vi "svx_SC Line Event Consumer.vi"(7 "shaft centerline":T2, 8 "State in":T3={"X Scale"={"Name"="Horizontal", "format string"="%#.2g", "Major Color"=16777238, "Minor Color"=16777216, "Scale Visible"=TRUE, " Label Visible"=TRUE, "Grid Style"=1, "Maximum"=1.0, "Minimum"=-1.0}, "Y Scale"={"Name"="Vertical", "format string"="%#.2g", "Major Color"=16777238, "Minor Color"=16777216, "Scale Visible"=TRUE, " Label Visible"=TRUE, "Grid Style"=1, "Maximum"=1.0, "Minimum"=-1.0}, "Plot"={"Point Style"=0, "Line Width"=0, "Line Style"=0, "Plot Color"=16860, "Point/fill"=16860}, "Arrow Color"=16860, "Autoscale"=TRUE, "Property Name"=[], "Container Bounds"={"Width"=550, "Height"=313}, "Background color"=16777226, "Annotation List"=[], "Cursor"={"Cursor Point Style"=13, "Cursor Style"=4, "Cursor Line Width"=1, "Cursor Line Style"=0, "Cursor Color"=16711680, "Cursor Name Visible"=TRUE, "Cursor Visible"=TRUE, "Cursor Position"={"X"=0.0, "Y"=0.0}, "Cursor Index"=0, "Lock Cursor Name"=FALSE, "Cursor reference"=0.0}, "size"=0, "Boundary Color"=9868950, "Maximum"=1.0, "Marker Point Style"=2, "Maker Visible"=TRUE, "Marker Color"=16860, "pair strings []"=[], "clearance boundary"=[{"boundary"={"x axis"=0.0, "y axis"=0.0}, "start point"=enum."center"}], "Custom pair name"=FALSE, "selector.visible"=TRUE, "Cursor Release"=refnum, "Children Tags"=[], "open?"=TRUE, "pair index"=[], "Legend Width"=200, " Parents Tags"="", "Label"="", "Legend Background"=16777226, "Legend Font"=16777222, "scale fit"=2, "user strings []"=[], "Item Width"=0, "out of state queue"=refnum, "property nodes"=refnum, "Kind"=enum."X-Scale", "Scale Range Change"=refnum} caption="State" {"pair index" min=0}, 10 "events":T7[](array[typedef]), 11 "references":T1) -> (0 "State out":T3={"X Scale"={"Name"="Horizontal", "format string"="%#.2g", "Major Color"=16777238, "Minor Color"=16777216, "Scale Visible"=TRUE, " Label Visible"=TRUE, "Grid Style"=1, "Maximum"=1.0, "Minimum"=-1.0}, "Y Scale"={"Name"="Vertical", "format string"="%#.2g", "Major Color"=16777238, "Minor Color"=16777216, "Scale Visible"=TRUE, " Label Visible"=TRUE, "Grid Style"=1, "Maximum"=1.0, "Minimum"=-1.0}, "Plot"={"Point Style"=0, "Line Width"=0, "Line Style"=0, "Plot Color"=16860, "Point/fill"=16860}, "Arrow Color"=16860, "Autoscale"=TRUE, "Property Name"=[], "Container Bounds"={"Width"=550, "Height"=313}, "Background color"=16777226, "Annotation List"=[], "Cursor"={"Cursor Point Style"=13, "Cursor Style"=4, "Cursor Line Width"=1, "Cursor Line Style"=0, "Cursor Color"=16711680, "Cursor Name Visible"=TRUE, "Cursor Visible"=TRUE, "Cursor Position"={"X"=0.0, "Y"=0.0}, "Cursor Index"=0, "Lock Cursor Name"=FALSE, "Cursor reference"=0.0}, "size"=0, "Boundary Color"=9868950, "Maximum"=1.0, "Marker Point Style"=2, "Maker Visible"=TRUE, "Marker Color"=16860, "pair strings []"=[], "clearance boundary"=[{"boundary"={"x axis"=0.0, "y axis"=0.0}, "start point"=enum."center"}], "Custom pair name"=FALSE, "selector.visible"=TRUE, "Cursor Release"=refnum, "Children Tags"=[], "open?"=TRUE, "pair index"=[], "Legend Width"=200, " Parents Tags"="", "Label"="", "Legend Background"=16777226, "Legend Font"=16777222, "scale fit"=2, "user strings []"=[], "Item Width"=0, "out of state queue"=refnum, "property nodes"=refnum, "Kind"=enum."X-Scale", "Scale Range Change"=refnum} caption="State" {"pair index" min=0})   [LabVIEW 2017, in "SVX SC Line.xctl"]
uses:
  <vilib>/addons/_XControls/Shaft Centerline/SVX SC Line.xctl
  <vilib>/addons/_XControls/Shaft Centerline/subVIs/svx_SC Line Core States.ctl
  <vilib>/addons/_XControls/Shaft Centerline/subVIs/svx_SC Line State.ctl
  <vilib>/addons/_XControls/Shaft Centerline/subVIs/svx_SC Line Bounds.ctl
  <vilib>/addons/_XControls/Shaft Centerline/subVIs/svx_SC Line Annotation List.ctl
  <vilib>/addons/_XControls/Shaft Centerline/subVIs/svx_SC Line OutState Queue.ctl
  <vilib>/addons/_XControls/Shaft Centerline/subVIs/svx_SC Line Data.ctl
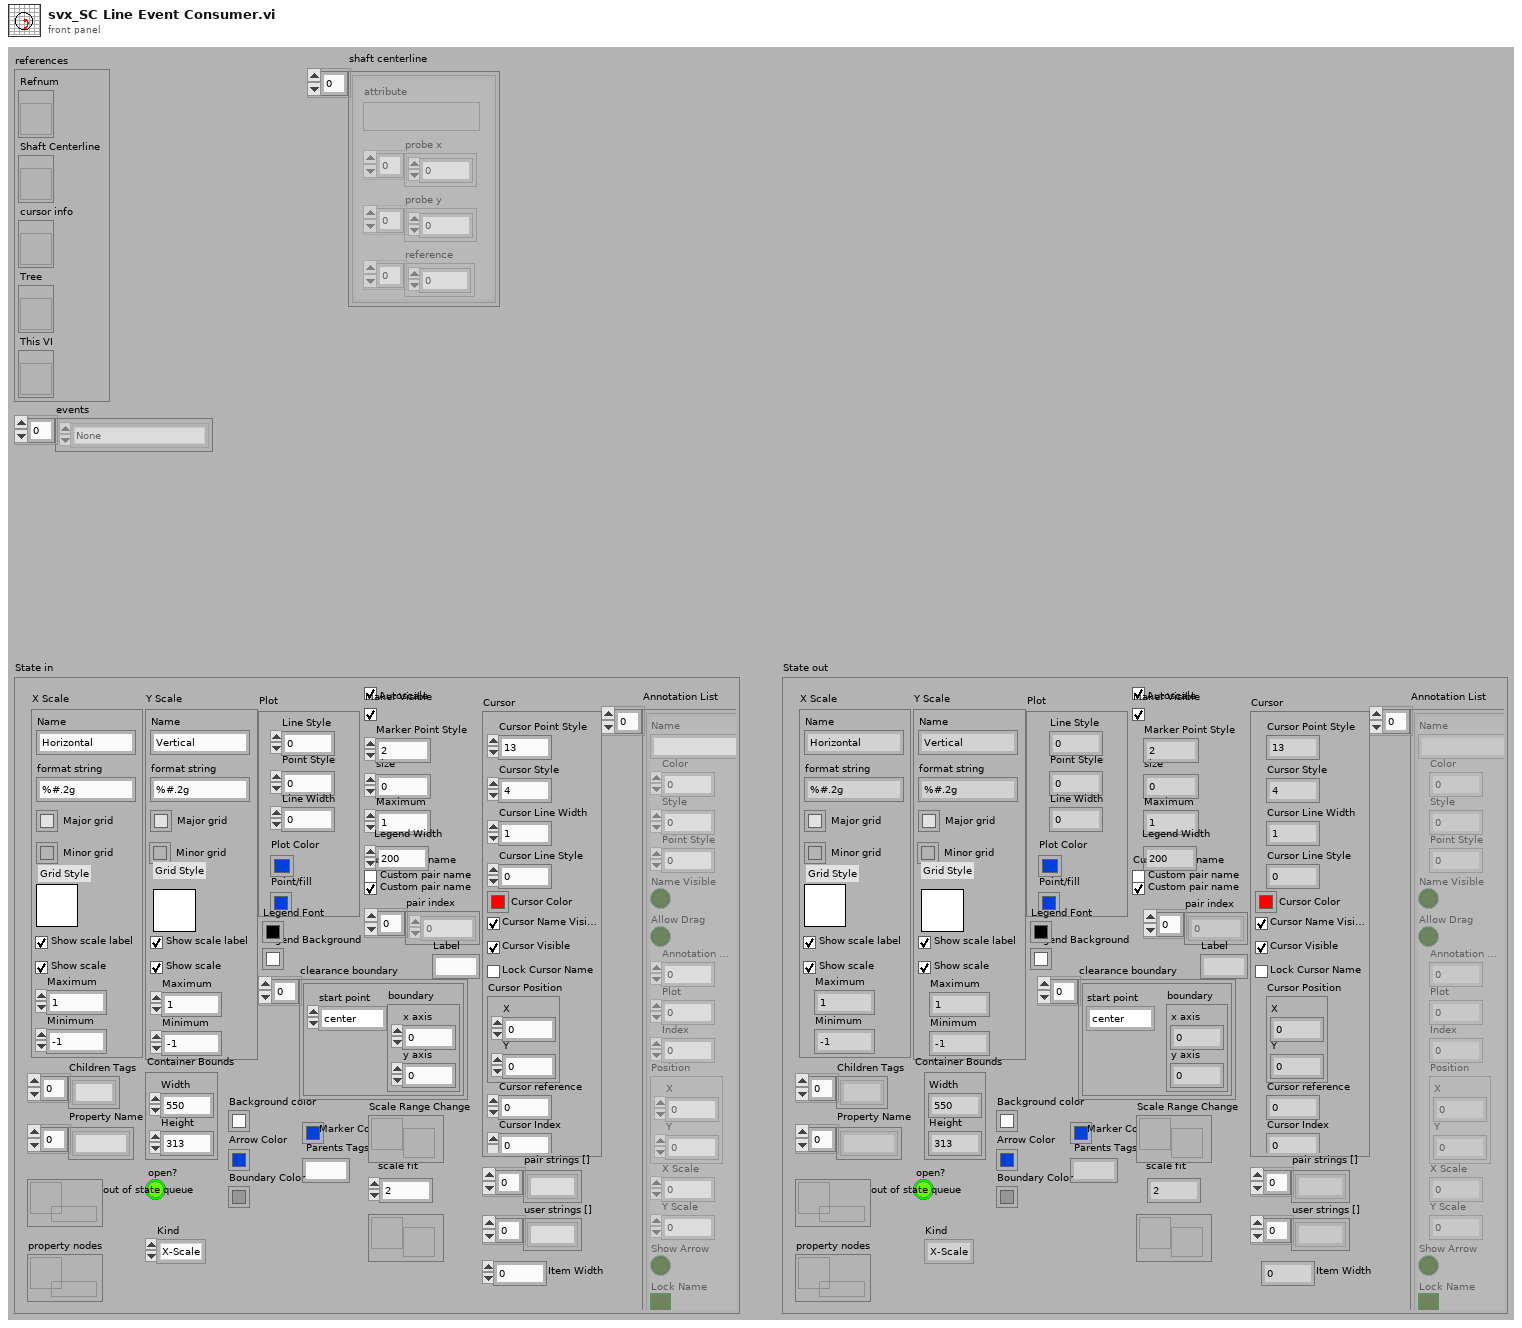
[diagram p1: front panel]
types:
  T1 = cluster{"Refnum":refnum<vi>, "Shaft Centerline":refnum<vi>, "cursor info":refnum<vi>, "Tree":refnum<vi>, "This VI":refnum<vi>}
  T2 = typedef "SVX SC Line.xctl/svx_SC Line Data.ctl" = cluster{"probe x":dbl[], "probe y":dbl[], "reference":dbl[], "attribute":variant}[]
  T3 = typedef "SVX SC Line.xctl/svx_SC Line State.ctl" = cluster{"X Scale":cluster{"Name":string, "format string":string, "Major Color":u32, "Minor Color":u32, "Scale Visible":bool, " Label Visible":bool, "Grid Style":u16, "Maximum":dbl, "Minimum":dbl}, "Y Scale":cluster{"Name":string, "format string":string, "Major Color":u32, "Minor Color":u32, "Scale Visible":bool, " Label Visible":bool, "Grid Style":u16, "Maximum":dbl, "Minimum":dbl}, "Plot":cluster{"Point Style":u8, "Line Width":u8, "Line Style":u8, "Plot Color":u32, "Point/fill":u32}, "Arrow Color":u32, "Autoscale":bool, "Property Name":string[], "Container Bounds":T4, "Background color":u32, "Annotation List":T5, "Cursor":cluster{"Cursor Point Style":u8, "Cursor Style":u8, "Cursor Line Width":u8, "Cursor Line Style":u8, "Cursor Color":u32, "Cursor Name Visible":bool, "Cursor Visible":bool, "Cursor Position":cluster{"X":dbl, "Y":dbl}, "Cursor Index":i32, "Lock Cursor Name":bool, "Cursor reference":dbl}, "size":i32, "Boundary Color":u32, "Maximum":dbl, "Marker Point Style":u8, "Maker Visible":bool, "Marker Color":u32, "pair strings []":string[], "clearance boundary":cluster{"boundary":cluster{"x axis":dbl, "y axis":dbl}, "start point":enum16{"center", "top", "bottom"}}[], "Custom pair name":bool, "selector.visible":bool, "Cursor Release":refnum<user-event>, "Children Tags":string[], "open?":bool, "pair index":i32[], "Legend Width":u32, " Parents Tags":string, "Label":string, "Legend Background":u32, "Legend Font":u32, "scale fit":u8, "user strings []":string[], "Item Width":u32, "out of state queue":T6, "property nodes":refnum<queue>, "Kind":enum16{"X-Scale", "Y-Scale", "Z-Scale"}, "Scale Range Change":refnum<user-event>}
  T4 = typedef "SVX SC Line.xctl/svx_SC Line Bounds.ctl" = cluster{"Width":u32, "Height":u32}
  T5 = typedef "SVX SC Line.xctl/svx_SC Line Annotation List.ctl" = cluster{"Name":string, "Color":u32, "Style":u8, "Point Style":u8, "Name Visible":bool, "Allow Drag":bool, "Annotation Mode":u32, "Plot":i32, "Index":i32, "Position":cluster{"X":dbl, "Y":dbl}, "X Scale":u32, "Y Scale":u32, "Show Arrow":bool, "Lock Name":bool, "Plot Area":i32, "Label Offset":cluster{"X":dbl, "Y":dbl}}[]
  T6 = typedef "SVX SC Line.xctl/svx_SC Line OutState Queue.ctl" = refnum<queue>
  T7 = typedef "SVX SC Line.xctl/svx_SC Line Core States.ctl" = enum16{"None", "[Axis] Autoscale", "[Image] Update", "[Cursor] Name", "[Plot] Grid&BG", "[Marker] Update", "[Tree] Tags", "[Data] Update", "[Layout] Size", "[Tree] Checkbox", "[Tree] Visible", "[Tree] Open", "[Axis] X", "[Axis] Y", "[Plot] Color", "[Axis] Format String", "[Data] Compare Strings", "[Cursor] Apearance", "[Axis] Name&Visible", "[Tree] Color", "[Data] Index", "[Cursor] Index", "[Axis] Event"}
  T8 = cluster{"X.Minimum":dbl, "X.Maximum":dbl, "Y.Minimum":dbl, "Y.Maximum":dbl, "Kind":enum16{"X-Scale", "Y-Scale", "Z-Scale"}}
  T9 = cluster{"boundary":cluster{"x axis":dbl, "y axis":dbl}, "start point":enum16{"center", "top", "bottom"}}[]
  T10 = cluster{"probe x":dbl[], "probe y":dbl[], "reference":dbl[], "attribute":variant}
  T11 = cluster{"boundary":cluster{"x axis":dbl, "y axis":dbl}, "start point":enum16{"center", "top", "bottom"}}
  T12 = cluster{"Cursor Point Style":u8, "Cursor Style":u8, "Cursor Line Width":u8, "Cursor Line Style":u8, "Cursor Color":u32, "Cursor Name Visible":bool, "Cursor Visible":bool, "Cursor Position":cluster{"X":dbl, "Y":dbl}, "Cursor Index":i32, "Lock Cursor Name":bool, "Cursor reference":dbl}
  T13 = typedef "LVPointDoubleTypeDef.ctl" = cluster{"Cursor X":dbl, "Cursor Y":dbl}
  T14 = cluster{"use queue?":bool, "Legend Width":u32, "Cursor reference":dbl, "Cursor Position":cluster{"X":dbl, "Y":dbl}, "pair strings []":string[], "Label":string, "Parents Tags":string, "Children Tags":string[], "Item Width":u32, "Maximum":dbl, "Minimum":dbl, "Maximum":dbl, "Minimum":dbl, "selector.visible":bool, "clearance boundary":cluster{"boundary":cluster{"x axis":dbl, "y axis":dbl}, "start point":enum16{"center", "top", "bottom"}}[], "size":i32}
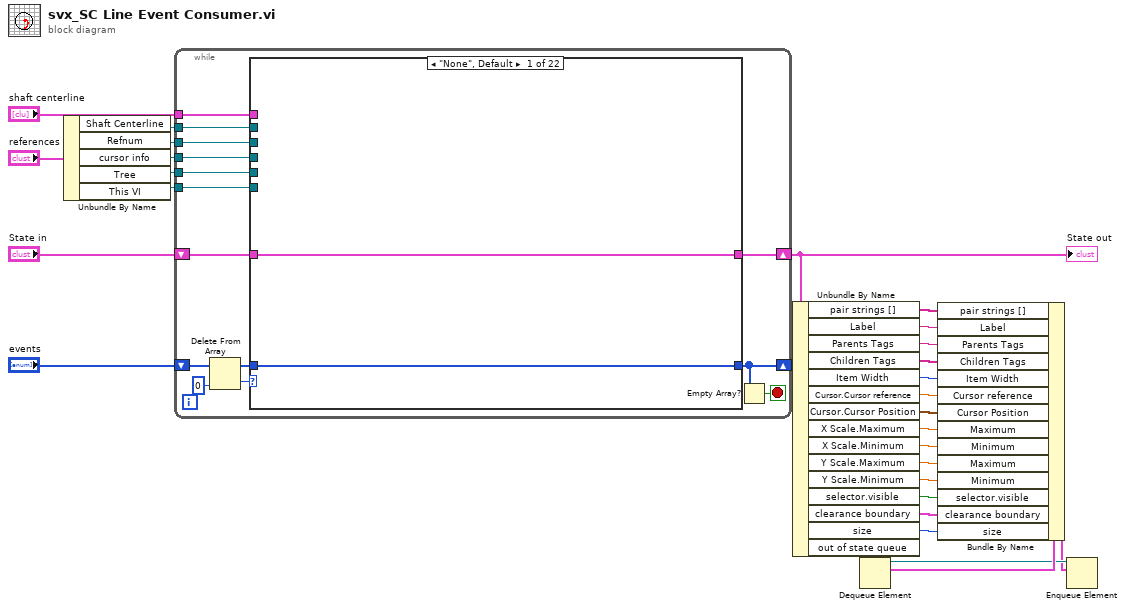
[diagram p0: block diagram]
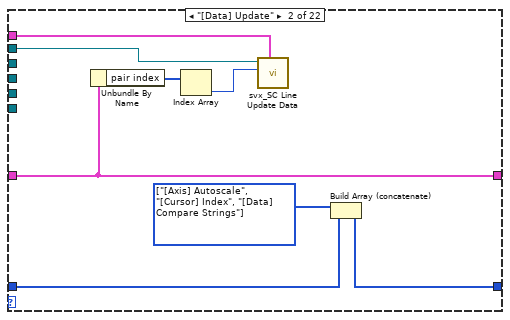
[diagram p2: hidden frame]
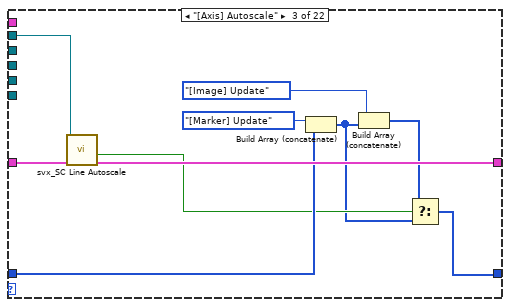
[diagram p3: hidden frame]
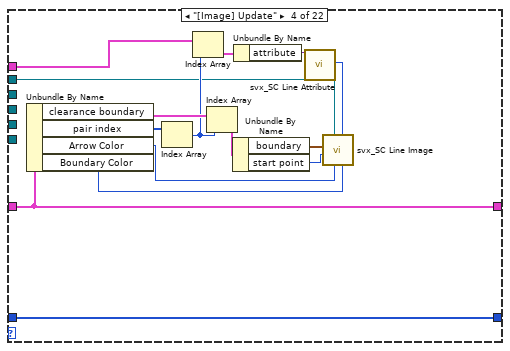
[diagram p4: hidden frame]
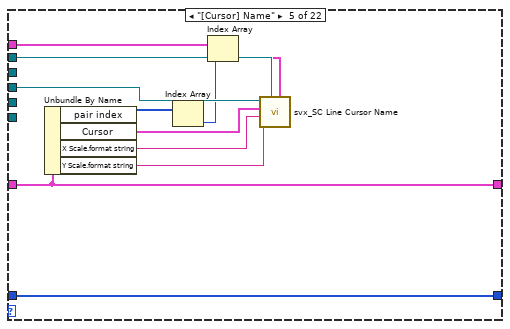
[diagram p5: hidden frame]
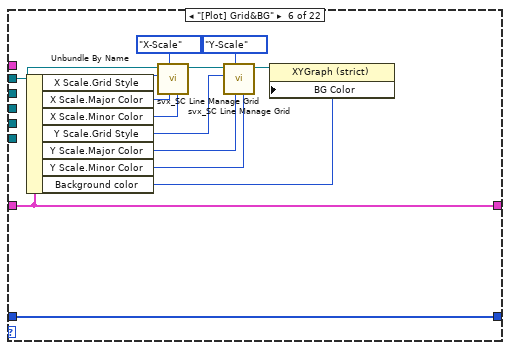
[diagram p6: hidden frame]
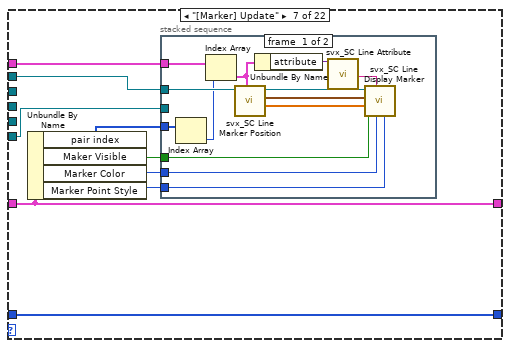
[diagram p7: hidden frame]
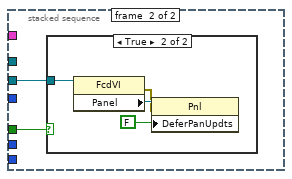
[diagram p8: hidden frame]
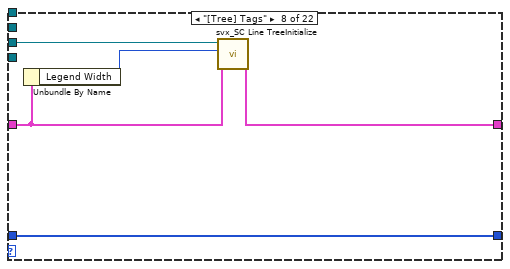
[diagram p10: hidden frame]
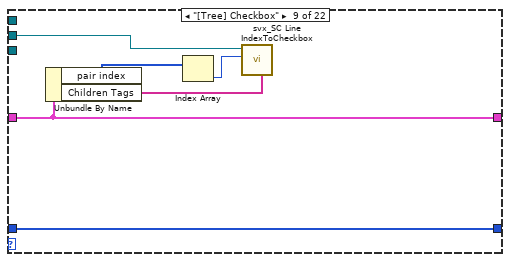
[diagram p11: hidden frame]
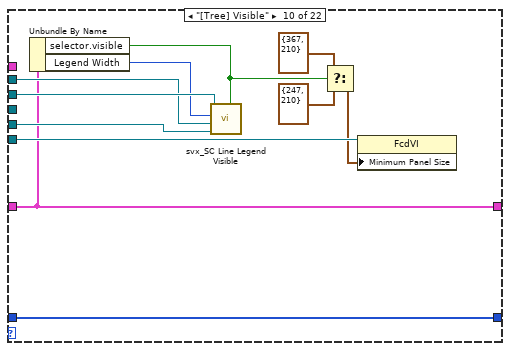
[diagram p12: hidden frame]
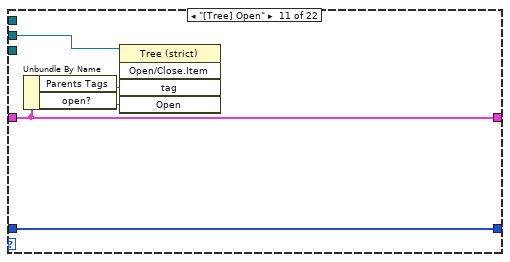
[diagram p13: hidden frame]
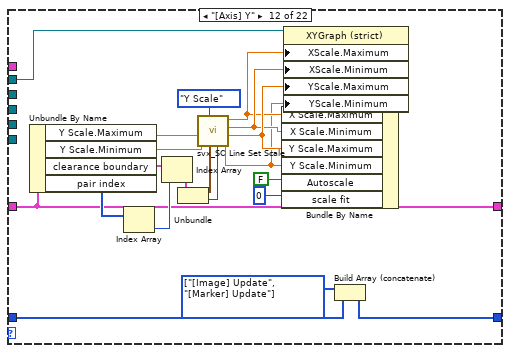
[diagram p14: hidden frame]
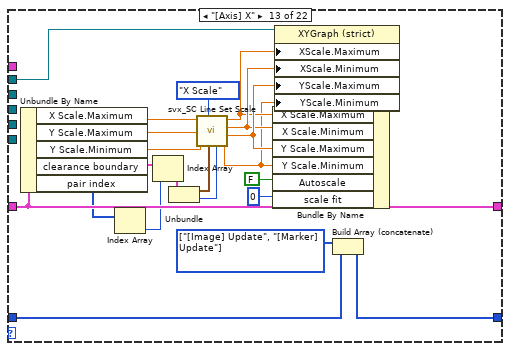
[diagram p15: hidden frame]
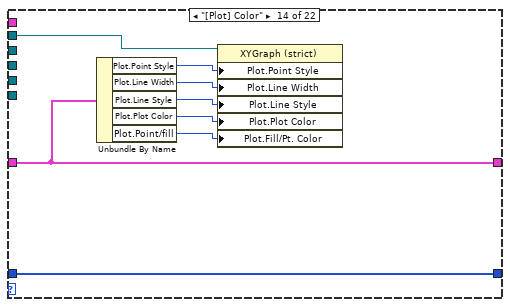
[diagram p16: hidden frame]
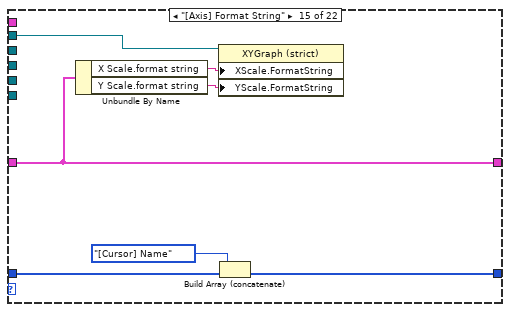
[diagram p17: hidden frame]
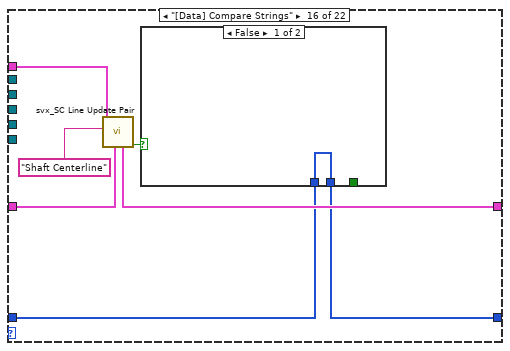
[diagram p18: hidden frame]
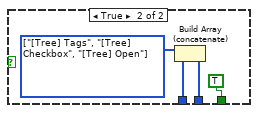
[diagram p19: hidden frame]
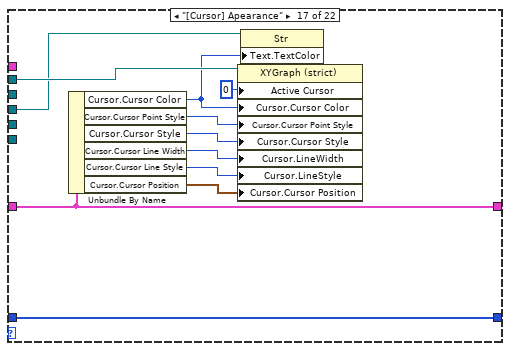
[diagram p20: hidden frame]
diagram:
  n1 = Unbundle By Name("references") -> ("Shaft Centerline"=w26:refnum<vi>, "Refnum"=w23:refnum<vi>, "cursor info"=w25:refnum<vi>, "Tree"=w24:refnum<vi>, "This VI"=w21:refnum<vi>)
  n2 = while {
    shift-right: [w42] -> w8
    shift-left: "State in" -> [w30]
    shift-right: [w36] -> _
    shift-left: "events" -> [w41]
    tunnel: "shaft centerline" -> [w35]
    tunnel: w26 -> [w34]
    tunnel: w25 -> [w33]
    tunnel: w24 -> [w32]
    tunnel: w23 -> [w31]
    tunnel: w21 -> [w29]
    stop <- w37 stop-if-true
    n3 = Delete From Array(array=w41, index=0) -> (deleted portion=w39:T7, array with subset deleted=w38:T7[])  [unwired: 1 in]
    n4 = case shown="\"None\", Default" w39 {
      tunnel: [w44 w50 w61 w77 w88 w93 w110 w135 w140 w142 w153 w166 w194 w202 w212 w221 w231 w247 w249 w264 w284 w292] -> w42
      tunnel: w38 -> [w43 w46 w58 w64 w78 w91 w104 w133 w136 w149 w154 w160 w181 w201 w210 w219 w230 w239 w248 w256 w286 w291]
      tunnel: [w43 w45 w59 w64 w78 w91 w104 w133 w136 w149 w154 w159 w180 w201 w209 w218 w230 w239 w248 w255 w285 w291] -> w36
      tunnel: w35 -> [_ w52 _ w67 w80 _ w105 _ _ _ _ _ _ _ _ w220 _ _ _ w274 _ _]
      tunnel: w34 -> [_ w51 w60 w63 w84 w92 w107 _ _ w151 _ w163 w192 w208 w215 _ w237 w246 _ w269 _ _]
      tunnel: w33 -> [_ _ _ _ w83 _ _ _ _ _ _ _ _ _ _ _ w229 _ _ _ _ _]
      tunnel: w32 -> [_ _ _ _ _ _ _ w134 w137 w150 w157 _ _ _ _ _ _ _ w252 _ _ _]
      tunnel: w31 -> [_ _ _ _ _ _ _ _ _ w152 _ _ _ _ _ _ _ _ _ _ _ _]
      tunnel: w30 -> [w44 w50 w62 w77 w88 w93 w110 w132 w140 w142 w153 w165 w193 w202 w212 w222 w231 w247 w249 w265 w284 w292]
      tunnel: w29 -> [_ _ _ _ _ _ w103 _ _ w146 _ _ _ _ _ _ _ _ _ _ _ _]
      frame "None", Default {
      }
      frame "[Data] Update" {
        w47 = T7[] [enum."[Axis] Autoscale", enum."[Cursor] Index", enum."[Data] Compare Strings"] items=["None", "[Axis] Autoscale", "[Image] Update", "[Cursor] Name", "[Plot] Grid&BG", "[Marker] Update", "[Tree] Tags", "[Data] Update", "[Layout] Size", "[Tree] Checkbox", "[Tree] Visible", "[Tree] Open", "[Axis] X", "[Axis] Y", "[Plot] Color", "[Axis] Format String", "[Data] Compare Strings", "[Cursor] Apearance", "[Axis] Name&Visible", "[Tree] Color", "[Data] Index", "[Cursor] Index", "[Axis] Event"] ("array")
        n5 = Unbundle By Name(w50) -> ("pair index"=w49:i32[])
        n6 = Index Array(array=w49) -> (element=w48:i32)  [unwired: 1 in]
        n7 = call <vilib>:"svx_SC Line Update Data.vi"("shaft centerline"=w52, "index"=w48, "reference"=w51) -> ()  [unwired: 9 in]
        n8 = Build Array (concatenate)(w47, w46) -> (w45:T7[])
      }
      frame "[Axis] Autoscale" {
        n9 = call <vilib>:"svx_SC Line Autoscale.vi"("State In"=w62, "SC Line in"=w60) -> ("State Out"=w61:T3, "use queue?"=w57:bool)  [unwired: 7 in, 1 out]
        n10 = Build Array (concatenate)(svx_SC_Line_Core_States."[Marker] Update" ("Property Page User Events"), w58) -> (w56:T7[])
        n11 = Build Array (concatenate)(svx_SC_Line_Core_States."[Image] Update" ("Property Page User Events"), w56) -> (w53:T7[])
        n12 = Select(t=w53, s=w57, f=w56) -> (s? t:f=w59:T7[])
      }
      frame "[Image] Update" {
        n13 = Unbundle By Name(w77) -> ("clearance boundary"=w72:T9, "pair index"=w69:i32[], "Arrow Color"=w76:u32, "Boundary Color"=w75:u32)
        n14 = Index Array(array=w69) -> (element=w66:i32)  [unwired: 1 in]
        n15 = Index Array(array=w67, index=w66) -> (element=w65:T10)
        n16 = Index Array(array=w72, index=w66) -> (element=w68:T11)
        n17 = Unbundle By Name(w68) -> ("boundary"=w71:cluster{"x axis":dbl, "y axis":dbl}, "start point"=w70:enum16{"center", "top", "bottom"})
        n18 = Unbundle By Name(w65) -> ("attribute"=w74:variant)
        n19 = call <vilib>:"svx_SC Line Attribute.vi"("attribute"=w74) -> ("rotating direction"=w73:u16)  [unwired: 14 in, 4 out]
        n20 = call <vilib>:"svx_SC Line Image.vi"("Boundary Color"=w75, "shaft rotating direction"=w73, "Arrow Color"=w76, "SC Line in"=w63, "start point"=w70, "boundary"=w71) -> ()  [unwired: 6 in]
      }
      frame "[Cursor] Name" {
        n21 = Unbundle By Name(w88) -> ("pair index"=w82:i32[], "Cursor"=w87:T12, "X Scale.format string"=w86:string, "Y Scale.format string"=w85:string)
        n22 = Index Array(array=w82) -> (element=w81:i32)  [unwired: 1 in]
        n23 = Index Array(array=w80, index=w81) -> (element=w79:T10)
        n24 = call <vilib>:"svx_SC Line Cursor Name.vi"("Data"=w79, "Shaft Centerline"=w84, "Y Scale.format string"=w85, "X Scale.format string"=w86, "Cursor"=w87, "cursor info"=w83) -> ()  [unwired: 6 in]
      }
      frame "[Plot] Grid&BG" {
        n25 = Unbundle By Name(w93) -> ("X Scale.Grid Style"=w99:u16, "X Scale.Major Color"=w98:u32, "X Scale.Minor Color"=w97:u32, "Y Scale.Grid Style"=w96:u16, "Y Scale.Major Color"=w95:u32, "Y Scale.Minor Color"=w94:u32, "Background color"=w89:u32)
        n26 = call <vilib>:"svx_SC Line Manage Grid.vi"("Minor Color"=w97, "Major Color"=w98, "Axis"=enum16{"X-Scale", "Y-Scale", "Z-Scale"}."X-Scale", "Grid Style"=w99, "Shaft Centerline in"=w92) -> ("Shaft Centerline out"=w102:refnum<vi>)  [unwired: 4 in, 2 out]
        n27 = call <vilib>:"svx_SC Line Manage Grid.vi"("Minor Color"=w94, "Major Color"=w95, "Axis"=enum16{"X-Scale", "Y-Scale", "Z-Scale"}."Y-Scale", "Grid Style"=w96, "Shaft Centerline in"=w102) -> ("Shaft Centerline out"=w90:refnum<vi>)  [unwired: 4 in, 2 out]
        n28 = property on="Property Node" class="XYGraph (strict)"(reference=w90, "BG Color"=w89) -> ()  [unwired: 1 in, 2 out]
      }
      frame "[Marker] Update" {
        n29 = Unbundle By Name(w110) -> ("pair index"=w106:i32[], "Maker Visible"=w108:bool, "Marker Color"=w111:u32, "Marker Point Style"=w109:u8)
        n30 = stacked-sequence {
          tunnel: w111 -> [w121 _]
          tunnel: w109 -> [w120 _]
          tunnel: w108 -> [w119 w125]
          tunnel: w107 -> [w116 _]
          tunnel: w106 -> [w115 _]
          tunnel: w105 -> [w114 _]
          tunnel: w103 -> [_ w126]
          frame #0 {
            n31 = Index Array(array=w115) -> (element=w113:i32)  [unwired: 1 in]
            n32 = Index Array(array=w114, index=w113) -> (element=w112:T10)
            n33 = call <vilib>:"svx_SC Line Marker Position.vi"("Data"=w112, "SC Line in"=w116) -> ("marker value"=w122:dbl[], "Marker Position"=w123:cluster{dbl, dbl}[], "SC Line out"=w124:refnum<vi>)  [unwired: 7 in]
            n34 = Unbundle By Name(w112) -> ("attribute"=w118:variant)
            n35 = call <vilib>:"svx_SC Line Attribute.vi"("attribute"=w118) -> ("x-axis selection"=w117:string)  [unwired: 14 in, 4 out]
            n36 = call <vilib>:"svx_SC Line Display Marker.vi"("Marker Style"=w120, "Marker Color"=w121, "time/rev/RPM"=w117, "Cursor.Visible"=w119, "Marker Values"=w122, "Marker Position"=w123, "Shaft Centerline"=w124) -> ()  [unwired: 5 in]
          }
          frame #1 {
            n37 = case shown="True" w125 {
              tunnel: w126 -> [_ w127]
              frame False {
              }
              frame True {
                n38 = property class="FcdVI"(reference=w127) -> (error out=w129:errorcluster, "Panel"=w130:refnum<vi>)  [unwired: 1 in, 1 out]
                n39 = property class="Pnl"(reference=w130, error in=w129, "DeferPanUpdts"=FALSE ("Defer Panel Updates")) -> ()  [unwired: 2 out]
              }
            }
          }
        }
      }
      frame "[Tree] Tags" {
        n40 = Unbundle By Name(w132) -> ("Legend Width"=w131:u32)
        n41 = call <vilib>:"svx_SC Line TreeInitialize.vi"("State in"=w132, "Legend Width"=w131, "Tree ref in"=w134) -> ("State out"=w135:T3)  [unwired: 7 in, 1 out]
      }
      frame "[Tree] Checkbox" {
        n42 = Unbundle By Name(w140) -> ("pair index"=w139:i32[], "Children Tags"=w141:string[])
        n43 = Index Array(array=w139) -> (element=w138:i32)  [unwired: 1 in]
        n44 = call <vilib>:"svx_SC Line IndexToCheckbox.vi"("All Children Tags"=w141, "RowIdx"=w138, "Tree ref in"=w137) -> ()  [unwired: 8 in, 1 out]
      }
      frame "[Tree] Visible" {
        n45 = Unbundle By Name(w142) -> ("selector.visible"=w143:bool, "Legend Width"=w144:u32)
        n46 = call <vilib>:"svx_SC Line Legend Visible.vi"("selector.visible"=w143, "Tree"=w150, "Shaft Centerline"=w151, "Legend Width"=w144, "container"=w152) -> ()  [unwired: 7 in]
        n47 = Select(t=cluster{"Horizontal":i16, "Vertical":i16} {"Horizontal"=367, "Vertical"=210} ("Front Panel Window:Minimum Size"), s=w143, f=cluster{"Horizontal":i16, "Vertical":i16} {"Horizontal"=247, "Vertical"=210}) -> (s? t:f=w145:cluster{"Horizontal":i16, "Vertical":i16})
        n48 = property class="FcdVI"(reference=w146, "Minimum Panel Size"=w145) -> ()  [unwired: 1 in, 2 out]
      }
      frame "[Tree] Open" {
        n49 = Unbundle By Name(w153) -> ("Parents Tags"=w156:string, "open?"=w155:bool)
        n50 = invoke on="Invoke Node" class="Tree (strict)" method="Open/Close.Item"(reference=w157, "tag"=w156, "Open"=w155) -> ()  [unwired: 2 in, 5 out]
      }
      frame "[Axis] Y" {
        w161 = T7[] [enum."[Image] Update", enum."[Marker] Update"] items=["None", "[Axis] Autoscale", "[Image] Update", "[Cursor] Name", "[Plot] Grid&BG", "[Marker] Update", "[Tree] Tags", "[Data] Update", "[Layout] Size", "[Tree] Checkbox", "[Tree] Visible", "[Tree] Open", "[Axis] X", "[Axis] Y", "[Plot] Color", "[Axis] Format String", "[Data] Compare Strings", "[Cursor] Apearance", "[Axis] Name&Visible", "[Tree] Color", "[Data] Index", "[Cursor] Index", "[Axis] Event"] ("array")
        n51 = Unbundle By Name(w165) -> ("Y Scale.Maximum"=w174:dbl, "Y Scale.Minimum"=w175:dbl, "clearance boundary"=w171:T9, "pair index"=w172:i32[])
        n52 = Index Array(array=w172) -> (element=w170:i32)  [unwired: 1 in]
        n53 = Index Array(array=w171, index=w170) -> (element=w169:T11)
        n54 = Unbundle(w169) -> ("boundary"=w168:cluster{"x axis":dbl, "y axis":dbl}, "start point"=w167:enum16{"center", "top", "bottom"})
        n55 = call <vilib>:"svx_SC Line Set Scale.vi"("start point"=w167, "boundary"=w168, "Selection"=enum16{"Autoscale", "X Scale", "Y Scale"}."Y Scale", "Y Min"=w175, "Y Max"=w174) -> ("Y Minimum"=w164:dbl, "Y Maximum"=w178:dbl, "X Minimum"=w177:dbl, "X Maximum"=w176:dbl)  [unwired: 3 in]
        n56 = Bundle By Name(cluster=w165, "X Scale.Maximum"=w176, "X Scale.Minimum"=w177, "Y Scale.Maximum"=w178, "Y Scale.Minimum"=w164, "Autoscale"=FALSE, "scale fit"=u8 0) -> (w166:T3)
        n57 = property on="Property Node" class="XYGraph (strict)"(reference=w163, "XScale.Maximum"=w176, "XScale.Minimum"=w177, "YScale.Maximum"=w178, "YScale.Minimum"=w164) -> ()  [unwired: 1 in, 2 out]
        n58 = Build Array (concatenate)(w161, w160) -> (w159:T7[])
      }
      frame "[Axis] X" {
        w182 = T7[] [enum."[Image] Update", enum."[Marker] Update"] items=["None", "[Axis] Autoscale", "[Image] Update", "[Cursor] Name", "[Plot] Grid&BG", "[Marker] Update", "[Tree] Tags", "[Data] Update", "[Layout] Size", "[Tree] Checkbox", "[Tree] Visible", "[Tree] Open", "[Axis] X", "[Axis] Y", "[Plot] Color", "[Axis] Format String", "[Data] Compare Strings", "[Cursor] Apearance", "[Axis] Name&Visible", "[Tree] Color", "[Data] Index", "[Cursor] Index", "[Axis] Event"] ("array")
        n59 = Unbundle By Name(w193) -> ("X Scale.Maximum"=w185:dbl, "Y Scale.Maximum"=w196:dbl, "Y Scale.Minimum"=w197:dbl, "clearance boundary"=w190:T9, "pair index"=w191:i32[])
        n60 = Index Array(array=w191) -> (element=w189:i32)  [unwired: 1 in]
        n61 = Index Array(array=w190, index=w189) -> (element=w188:T11)
        n62 = Unbundle(w188) -> ("boundary"=w187:cluster{"x axis":dbl, "y axis":dbl}, "start point"=w186:enum16{"center", "top", "bottom"})
        n63 = call <vilib>:"svx_SC Line Set Scale.vi"("start point"=w186, "boundary"=w187, "Selection"=enum16{"Autoscale", "X Scale", "Y Scale"}."X Scale", "Y Min"=w197, "Y Max"=w196, "X Max"=w185) -> ("Y Minimum"=w184:dbl, "Y Maximum"=w200:dbl, "X Minimum"=w199:dbl, "X Maximum"=w198:dbl)  [unwired: 2 in]
        n64 = Bundle By Name(cluster=w193, "X Scale.Maximum"=w198, "X Scale.Minimum"=w199, "Y Scale.Maximum"=w200, "Y Scale.Minimum"=w184, "Autoscale"=FALSE, "scale fit"=u8 0) -> (w194:T3)
        n65 = property on="Property Node" class="XYGraph (strict)"(reference=w192, "XScale.Maximum"=w198, "XScale.Minimum"=w199, "YScale.Maximum"=w200, "YScale.Minimum"=w184) -> ()  [unwired: 1 in, 2 out]
        n66 = Build Array (concatenate)(w182, w181) -> (w180:T7[])
      }
      frame "[Plot] Color" {
        n67 = Unbundle By Name(w202) -> ("Plot.Point Style"=w207:u8, "Plot.Line Width"=w206:u8, "Plot.Line Style"=w205:u8, "Plot.Plot Color"=w204:u32, "Plot.Point/fill"=w203:u32)
        n68 = property on="Property Node" class="XYGraph (strict)"(reference=w208, "Plot.Point Style"=w207, "Plot.Line Width"=w206, "Plot.Line Style"=w205, "Plot.Plot Color"=w204, "Plot.Fill/Pt. Color"=w203) -> ()  [unwired: 1 in, 2 out]
      }
      frame "[Axis] Format String" {
        n69 = Unbundle By Name(w212) -> ("X Scale.format string"=w214:string, "Y Scale.format string"=w213:string)
        n70 = property on="Property Node" class="XYGraph (strict)"(reference=w215, "XScale.FormatString"=w214, "YScale.FormatString"=w213) -> ()  [unwired: 1 in, 2 out]
        n71 = Build Array (concatenate)(svx_SC_Line_Core_States."[Cursor] Name" ("Property Page User Events"), w210) -> (w209:T7[])
      }
      frame "[Data] Compare Strings" {
        n72 = call <vilib>:"svx_SC Line Update Pair.vi"("State in"=w222, "Label.Text"="Shaft Centerline", "shaft centerline"=w220) -> ("update tree?"=w217:bool, "State out"=w221:T3)  [unwired: 7 in]
        n73 = case shown="False" w217 {
          tunnel: w219 -> [w223 w227]
          tunnel: [w223 w226] -> w218
          tunnel: [_ TRUE ("data changed?")] -> _
          frame False {
          }
          frame True {
            w225 = T7[] [enum."[Tree] Tags", enum."[Tree] Checkbox", enum."[Tree] Open"] items=["None", "[Axis] Autoscale", "[Image] Update", "[Cursor] Name", "[Plot] Grid&BG", "[Marker] Update", "[Tree] Tags", "[Data] Update", "[Layout] Size", "[Tree] Checkbox", "[Tree] Visible", "[Tree] Open", "[Axis] X", "[Axis] Y", "[Plot] Color", "[Axis] Format String", "[Data] Compare Strings", "[Cursor] Apearance", "[Axis] Name&Visible", "[Tree] Color", "[Data] Index", "[Cursor] Index", "[Axis] Event"] ("array")
            n74 = Build Array (concatenate)(w225, w227) -> (w226:T7[])
          }
        }
      }
      frame "[Cursor] Apearance" {
        n75 = Unbundle By Name(w231) -> ("Cursor.Cursor Color"=w228:u32, "Cursor.Cursor Point Style"=w236:u8, "Cursor.Cursor Style"=w235:u8, "Cursor.Cursor Line Width"=w234:u8, "Cursor.Cursor Line Style"=w233:u8, "Cursor.Cursor Position"=w232:cluster{"X":dbl, "Y":dbl})
        n76 = property on="Property Node" class="XYGraph (strict)"(reference=w237, "Active Cursor"=u32 0, "Cursor.Cursor Color"=w228, "Cursor.Cursor Point Style"=w236, "Cursor.Cursor Style"=w235, "Cursor.LineWidth"=w234, "Cursor.LineStyle"=w233, "Cursor.Cursor Position"=w232) -> ()  [unwired: 1 in, 2 out]
        n77 = property on="Property Node" class="Str"(reference=w229, "Text.TextColor"=w228) -> ()  [unwired: 1 in, 2 out]
      }
      frame "[Axis] Name&Visible" {
        n78 = Unbundle By Name(w247) -> ("X Scale.Name"=w245:string, "X Scale.Scale Visible"=w244:bool, "X Scale.Label Visible"=w243:bool, "Y Scale.Name"=w242:string, "Y Scale.Scale Visible"=w241:bool, "Y Scale.Label Visible"=w240:bool)
        n79 = property on="Property Node" class="XYGraph (strict)"(reference=w246, "XScale.NameLbl.Text"=w245, "XScale.Visible"=w244, "XScale.NameLbl.Visible"=w243, "YScale.NameLbl.Text"=w242, "YScale.Visible"=w241, "YScale.NameLbl.Visible"=w240) -> ()  [unwired: 1 in, 2 out]
      }
      frame "[Tree] Color" {
        w253 = -2 ("Active Cell:Active Column Number")
        n80 = Unbundle By Name(w249) -> ("Legend Background"=w251:u32, "Legend Font"=w250:u32)
        n81 = property on="Property Node" class="Tree (strict)"(reference=w252, "ActiveColNum"=w253, "Active Item Row Number"=w253, "CellBG"=w251, "CellFontColor"=w250) -> ()  [unwired: 1 in, 2 out]
      }
      frame "[Cursor] Index" {
        n82 = Unbundle By Name(w265) -> ("pair index"=w275:i32[], "Cursor.Cursor Index"=w268:i32, "Cursor.Cursor Position"=w262:cluster{"X":dbl, "Y":dbl}, "Cursor.Cursor reference"=w260:dbl)
        n83 = Index Array(array=w275) -> (element=w276:i32)  [unwired: 1 in]
        n84 = Index Array(array=w274, index=w276) -> (element=w273:T10)
        n85 = Unbundle(w273) -> ("reference"=w267:dbl[])  [unwired: 3 out]
        n86 = Array Size(array=w267) -> (size(s)=w272:i32)
        n87 = Decrement(x=w272) -> (x-1=w271:i32)
        n88 = property on="Property Node" class="XYGraph (strict)"(reference=w269, "Active Cursor"=u32 0, "Cursor.Cursor Index"=w268) -> ("Cursor.Cursor Position"=w263:T13)  [unwired: 1 in, 2 out]
        n89 = In Range and Coerce(upper limit=w271, x=w268, lower limit=0) -> (coerced(x)=w266:i32)  [unwired: 1 out]
        n90 = Build Array (concatenate)(svx_SC_Line_Core_States."[Cursor] Name" ("Property Page User Events"), w256) -> (w255:T7[])
        n91 = Index Array(array=w267, index=w266) -> (element=w261:dbl)
        n92 = Not Equal?(x=w263, y=w262) -> (x != y?=w259:bool)
        n93 = Not Equal?(x=w261, y=w260) -> (x != y?=w258:bool)
        n94 = Or(x=w259, y=w258) -> (x .or. y?=w257:bool)
        n95 = case shown="True" w257 {
          tunnel: w265 -> [w278 w283]
          tunnel: [w278 w282] -> w264
          tunnel: w263 -> [_ w281]
          tunnel: w261 -> [_ w280]
          tunnel: [_ TRUE ("data changed?")] -> _
          frame False {
          }
          frame True {
            n96 = Bundle By Name(cluster=w283, "Cursor.Cursor Position"=w281, "Cursor.Cursor reference"=w280) -> (w282:T3)
          }
        }
      }
      frame "[Data] Index" {
        w287 = T7[] [enum."[Data] Update", enum."[Tree] Checkbox", enum."[Image] Update", enum."[Marker] Update"] items=["None", "[Axis] Autoscale", "[Image] Update", "[Cursor] Name", "[Plot] Grid&BG", "[Marker] Update", "[Tree] Tags", "[Data] Update", "[Layout] Size", "[Tree] Checkbox", "[Tree] Visible", "[Tree] Open", "[Axis] X", "[Axis] Y", "[Plot] Color", "[Axis] Format String", "[Data] Compare Strings", "[Cursor] Apearance", "[Axis] Name&Visible", "[Tree] Color", "[Data] Index", "[Cursor] Index", "[Axis] Event"] ("array")
        n97 = Build Array (concatenate)(w287, w286) -> (w285:T7[])
      }
      frame "[Axis] Event" {
        n98 = Unbundle By Name(w292) -> ("Scale Range Change"=w294:refnum<user-event>, "Kind"=w297:enum16{"X-Scale", "Y-Scale", "Z-Scale"}, "X Scale.Minimum"=w296:dbl, "X Scale.Maximum"=w295:dbl, "Y Scale.Minimum"=w289:dbl, "Y Scale.Maximum"=w288:dbl)
        n99 = Bundle By Name(cluster=T8 {"X.Minimum"=0.0, "X.Maximum"=0.0, "Y.Minimum"=0.0, "Y.Maximum"=0.0, "Kind"=enum."X-Scale"} ("output cluster"), "Kind"=w297, "X.Minimum"=w296, "X.Maximum"=w295, "Y.Minimum"=w289, "Y.Maximum"=w288) -> (w293:T8)
        n100 = Generate User Event(user event=w294, event data cluster=w293) -> ()  [unwired: 2 in, 2 out]
      }
    }
    n101 = Empty Array?(array=w36) -> (empty?=w37:bool)
  }
  "State out" <- w8
  n102 = Unbundle By Name(w8) -> ("pair strings []"=w18:string[], "Label"=w19:string, "Parents Tags"=w20:string, "Children Tags"=w17:string[], "Item Width"=w16:u32, "Cursor.Cursor reference"=w15:dbl, "Cursor.Cursor Position"=w14:cluster{"X":dbl, "Y":dbl}, "X Scale.Maximum"=w13:dbl, "X Scale.Minimum"=w12:dbl, "Y Scale.Maximum"=w11:dbl, "Y Scale.Minimum"=w10:dbl, "selector.visible"=w9:bool, "clearance boundary"=w7:T9, "size"=w1:i32, "out of state queue"=w5:T6)
  n103 = Dequeue Element(queue=w5) -> (queue out=w3:T6, element=w4:T14)  [unwired: 2 in, 2 out]
  n104 = Bundle By Name(cluster=w4, "pair strings []"=w18, "Label"=w19, "Parents Tags"=w20, "Children Tags"=w17, "Item Width"=w16, "Cursor reference"=w15, "Cursor Position"=w14, "Maximum"=w13, "Minimum"=w12, "Maximum"=w11, "Minimum"=w10, "selector.visible"=w9, "clearance boundary"=w7, "size"=w1) -> (w2:T14)
  n105 = Enqueue Element(queue=w3, element=w2) -> ()  [unwired: 2 in, 3 out]
